vi "construct lorentzian - V2.vi"(10 "omega  in":dbl[](array[numeric]), 11 "lorentzian":T1={"A (VHz)"=-1.0311345636926572, "f (Hz)"=-1.0311345636926572, "G (Hz)"=-1.0311345636926572, "phi(rad)"=-1.0311345636926572, "Q"=-1.0311345636926572, "Norm  Ampl"=-1.0311345636926572, "bg (V)"=-1.0311345636926572+0.0i, "4corners"={"z (-pi/2)"=-1.0311345636926572+0.5736824521422934i, "z(inf)"=-0.5200164984937075+1.0975277942502903i, "z (pi/2)"=-1.0311345636926572+0.5736824521422934i, "z center"=-0.5136528600391839+0.580046090596817i, "z(0)"=-0.5200164984937075+1.0975277942502903i, "radius"=-1.0311345636926572}} {"bg (V)" format="%#9_9f"; "Q" format="%#9_9f"; "phi(rad)" format="%#9_9f"; "G (Hz)" format="%#9_9f"; "f (Hz)" format="%#9_9f"}) -> (3 "z out":cdb[](array[numeric]))   [LabVIEW 2018]
uses:
  lorentzian.ctl
  circle corners.ctl
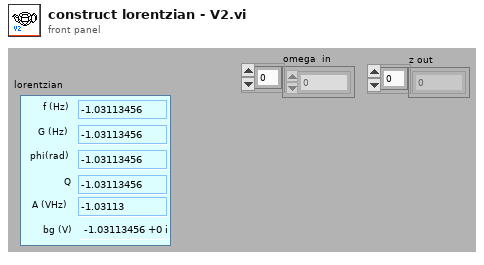
[diagram p1: front panel]
types:
  T1 = typedef "lorentzian.ctl" = cluster{"A (VHz)":dbl, "f (Hz)":dbl, "G (Hz)":dbl, "phi(rad)":dbl, "Q":dbl, "Norm  Ampl":dbl, "bg (V)":cdb, "4corners":T2}
  T2 = typedef "circle corners.ctl" = cluster{"z (-pi/2)":cdb, "z(inf)":cdb, "z (pi/2)":cdb, "z center":cdb, "z(0)":cdb, "radius":dbl}
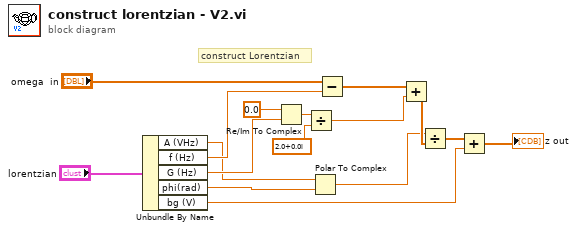
[diagram p0: block diagram]
diagram:
  # "construct Lorentzian"
  n1 = Unbundle By Name("lorentzian") -> ("A (VHz)"=w2:dbl, "f (Hz)"=w9:dbl, "G (Hz)"=w8:dbl, "phi(rad)"=w3:dbl, "bg (V)"=w4:cdb)
  n2 = Re/Im To Complex(1:w8, 2:0.0 ("x")) -> (0:w14:cdb)
  n3 = Divide(x=w14, y=cdb 2.0+0.0i) -> (x/y=w12:cdb)
  n4 = Polar To Complex(1:w3, 2:w2) -> (0:w1:cdb)
  n5 = Subtract(x="omega  in", y=w9) -> (x-y=w16:dbl[])
  n6 = Add(x=w16, y=w12) -> (x+y=w11:cdb[])
  n7 = Divide(x=w1, y=w11) -> (x/y=w10:cdb[])
  n8 = Add(x=w10, y=w4) -> (x+y=→"z out":cdb[])
